vi "dkalm.vi"() -> ()   [LabVIEW 2017]
uses:
  <vilib>/Analysis/Matrix/Datatypes/RealMatrix.ctl
  <vilib>/Analysis/Matrix/Numeric/Conversions/Array To Matrix - RA2.vi
  <vilib>/Analysis/Matrix/NI_Matrix.lvlib
panel:
  out "L":T1=[[0.0, 50.2704], [0.0, -0.0], [0.0, 0.0], [0.0, 0.0]]
  in  "Gains":T2={"A"=[[0.0, 1.0], [0.0, -50.28030731]], "B"=[], "C"=[[1.0, 0.0]], "D"=[], "Q"=[[0.05, 1.0]], "R"=[[0.0001]], "K"=[], "Kff"=[], "L"=[]}
  out "standard output":string="0.0000,50.2704\r\n0.0000,-0.0000\r\n[[      0.              -0.        ]\r\n [     -0.         3200095.15290555]]\r\n"
  out "standard error":string
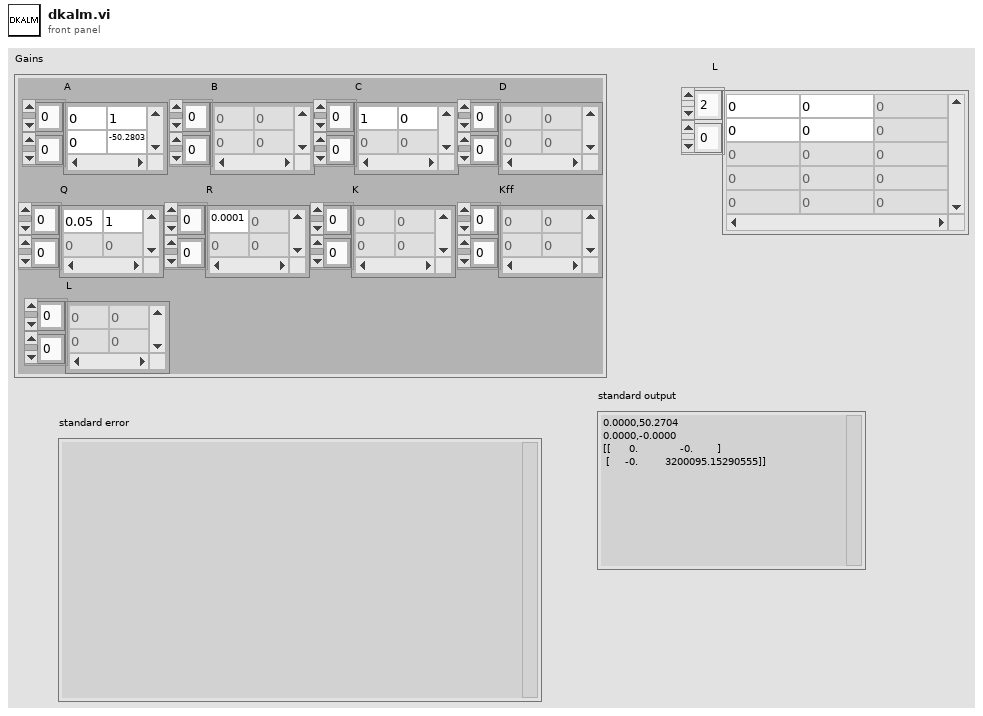
[diagram p1: front panel]
types:
  T1 = typedef "NI_Matrix.lvlib/RealMatrix.ctl" = dbl[][]
  T2 = cluster{"A":T1, "B":T1, "C":T1, "D":T1, "Q":T1, "R":T1, "K":T1, "Kff":T1, "L":T1}
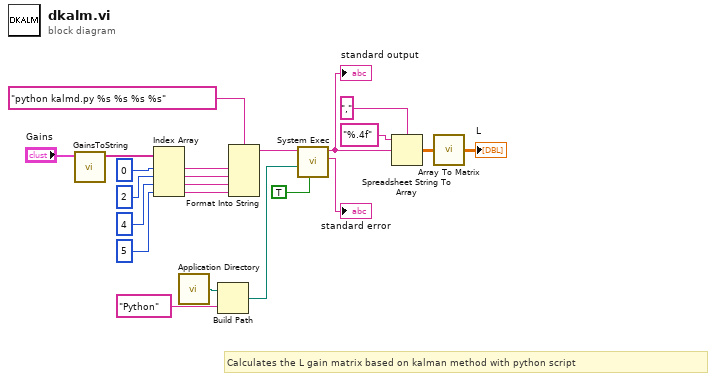
[diagram p0: block diagram]
diagram:
  # "Calculates the L gain matrix based on kalman method with python script"
  n1 = call "GainsToString.vi"("Gains"="Gains") -> ("Strings"=w14:string[])  [unwired: 10 in]
  n2 = Index Array(array=w14, index #1=0 ("index"), index #2=2 ("index"), index #3=4 ("index"), index #4=5 ("index")) -> (element #1=w13:string, element #2=w12:string, element #3=w9:string, element #4=w8:string)
  n3 = call <vilib>:"Application Directory.vi"() -> ("Application Directory"=w22:path)
  n4 = Build Path(base path=w22, name or relative path="Python") -> (appended path=w20:path)
  n5 = Format Into String(format string="python kalmd.py %s %s %s %s" ("command line"), w13, w12, w9, w8) -> (resulting string=w16:string)  [unwired: 2 in, 1 out]
  n6 = call <vilib>:"System Exec.vi"("run minimized? (F)"=TRUE, "working directory"=w20, "command line"=w16) -> ("standard error"=→"standard error":string, "standard output"=w3:string)  [unwired: 5 in, 2 out]
  "standard output" <- w3
  n7 = Spreadsheet String To Array(delimiter (Tab)=",", format string="%.4f", spreadsheet string=w3) -> (array=w2:dbl[][])  [unwired: 1 in]
  n8 = call-poly <vilib>:"Array To Matrix.vi"("Real 2D Array"=w2) -> ("Real Matrix"=→"L":T1)
